vi "VIAn_CheckBrokenVIs.vi"(8 "error in (no error)":errorcluster, 11 "CommandLine":string[](array[string])) -> (0 "error out":errorcluster, 2 "test details":string, 3 "output to action":string)   [LabVIEW 2014]
uses:
  <userlib>/_OpenG.lib/string/string.llb/Trim Whitespace (String)__ogtk.vi
  <userlib>/_OpenG.lib/file/file.llb/File Exists - Scalar__ogtk.vi
  <userlib>/_OpenG.lib/array/array.llb/Filter 1D Array with Scalar (String)__ogtk.vi
  <userlib>/_OpenG.lib/array/array.llb/Empty 1D Array (String)__ogtk.vi
  <userlib>/_OpenG.lib/file/file.llb/Compare Two Paths - Scalar__ogtk.vi
  _lvcicd/_lvcicd_support_2014.lvlib
  <vilib>/addons/analyzer/NI_VIAnalyzerTKVIs.lvlib
panel:
  out "Analysis Progress":dbl(slide) scale=0.0..100.0
  out "VI in Analysis":string
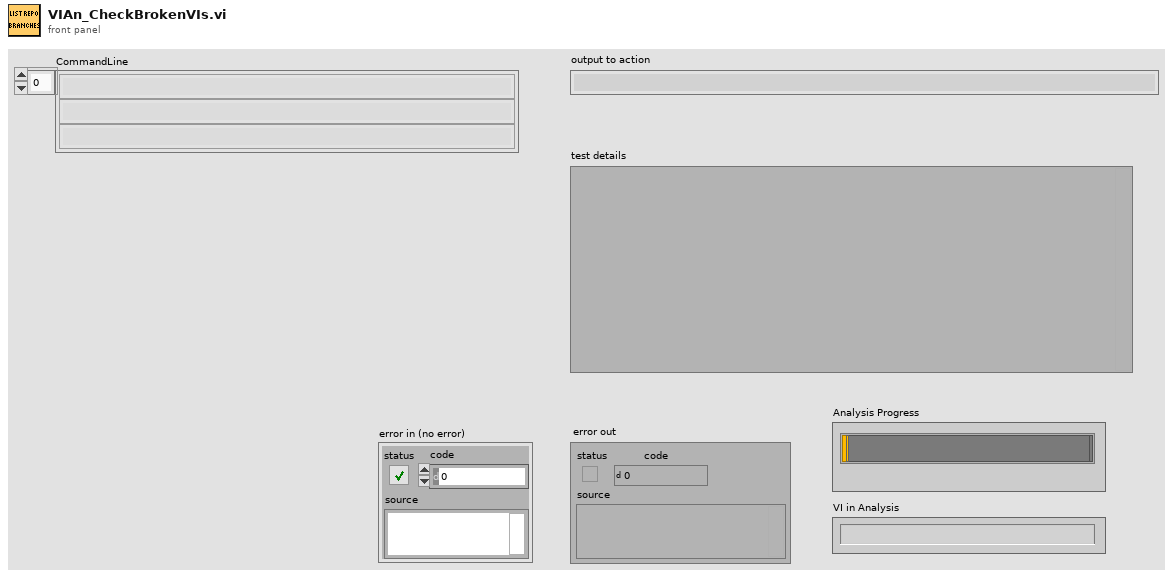
[diagram p1: front panel]
types:
  T1 = typedef "VIAnAPI Ref.ctl" = refnum<k1>
  T2 = typedef "VIAnCtl API Test Config Data.ctl" = cluster{"Test Ranking":T3, "Max Failures":u32, "Control Values":T4[], "Run Test?":bool}
  T3 = typedef "VIAnCtl TestRanking.ctl" = u16
  T4 = typedef "VIAnCtl Config Control Value.ctl" = cluster{"Control Name":string, "Control Value":variant}
  T5 = typedef "VIAnCtl Results.ctl" = cluster{"Test Name":string, "Results Data":T6[], "Status":T7, "Exceed Max Fails?":bool}
  T6 = typedef "VIAnCtl ResultsData (index).ctl" = cluster{"Result Message":string, "Ref Index":i32}
  T7 = typedef "VIAnCtl ResultStatus.ctl" = enum16{"Pass", "Fail", "Skipped", "VI not loadable", "Test not loadable", "Test not runnable", "Test error out"}
  T8 = typedef "VIAnRes Parsed Results Data (by VI).ctl" = cluster{"VI Path":path, "Pass":cluster{"row":i32, "column":i32}[], "Fail":cluster{"row":i32, "column":i32}[], "Skipped":cluster{"row":i32, "column":i32}[], "VI not loadable":cluster{"row":i32, "column":i32}[], "Test not loadable":cluster{"row":i32, "column":i32}[], "Test not runnable":cluster{"row":i32, "column":i32}[], "Test error out":cluster{"row":i32, "column":i32}[]}
  T9 = typedef "VIAnRes Parsed Results Data (by Test).ctl" = cluster{"Test Name":string, "Pass":cluster{"VI Path":path, "index":cluster{"row":i32, "column":i32}}[], "Fail":cluster{"VI Path":path, "index":cluster{"row":i32, "column":i32}}[], "Skipped":cluster{"VI Path":path, "index":cluster{"row":i32, "column":i32}}[]}
  T10 = typedef "VIAnCtl Test Config Data.ctl" = cluster{"Test Name":string, "Config Ref":refnum<vi>, "Ref Valid?":bool, "Test Ranking":T3, "Max Failures":u32, "Test Path":path, "Control Values":T4[], "Selected?":bool}
  T11 = cluster{"Raw Results":T5[][], "Parsed Results Data (by VI)":T8[], "Parsed Results Data (by Test)":T9[], "Summary Statistics":cluster{"Passed Tests":i32, "Failed Tests":i32, "Skipped Tests":i32, "VIs not loadable":i32, "Tests not loadable":i32, "Tests not runnable":i32, "Test error out":i32, "Start Time":u32, "Total Time (s)":dbl}, "Test Config Data":T10[]}
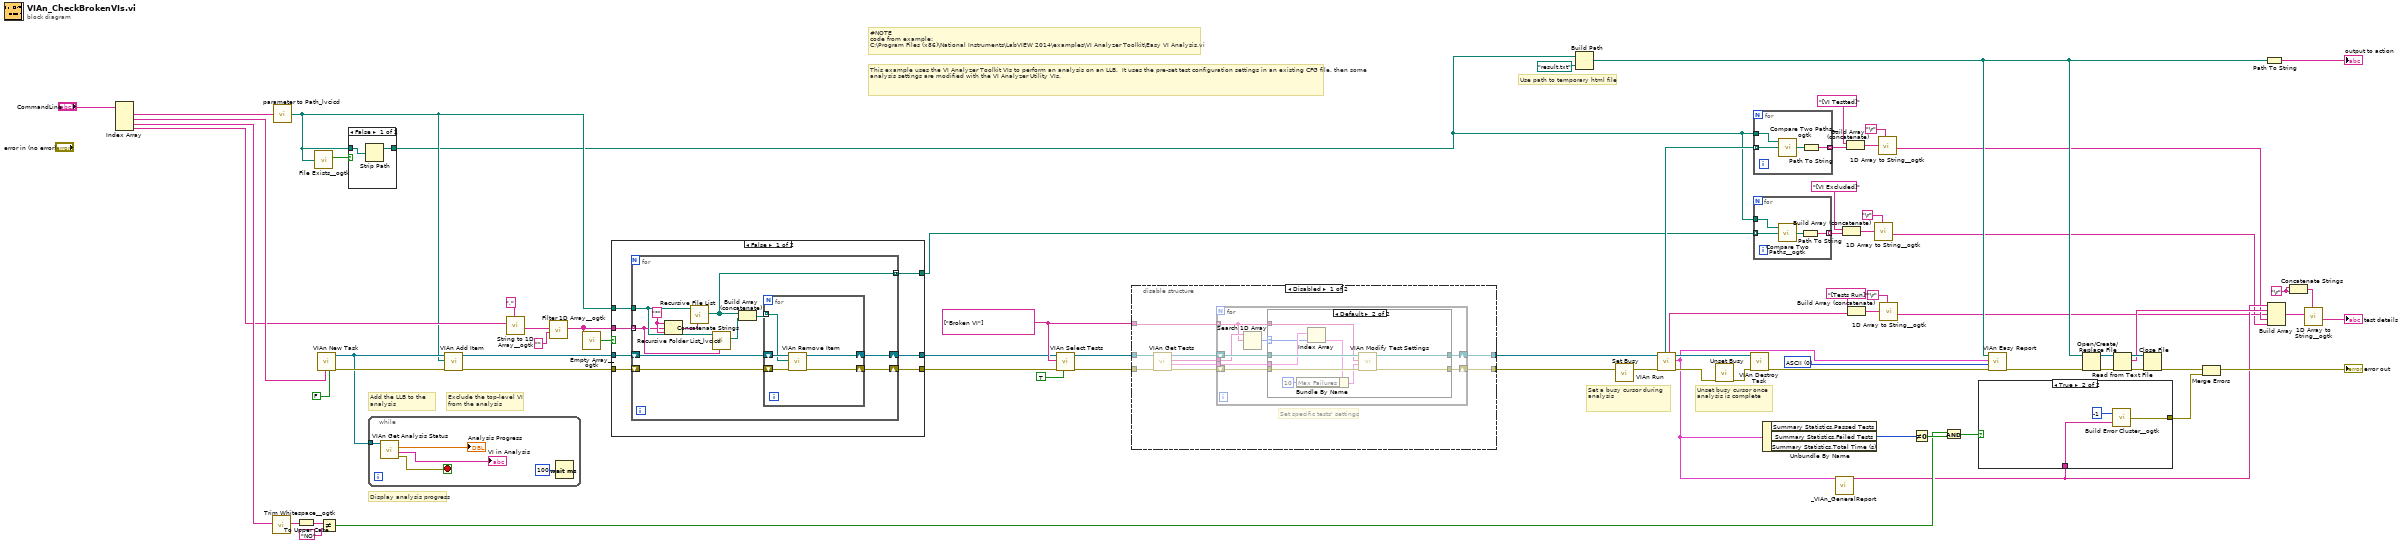
[diagram p0: block diagram]
diagram:
  w34 = "\r"
  w52 = string[] ["Broken VI"] ("Excluded Tests")
  w61 = u16 0 items=["ASCII", "HTML", "RSL File"] ("Report Save Type (ASCII)")
  # "Display analysis progress"
  # "Unset busy cursor once analysis is complete"
  # "Set a busy cursor during analysis"
  # "This example uses the VI Analyzer Toolkit VIs to perform an analysis on an LLB.  It uses the pre-set test configuration settings in an existing CFG file, then some analysis settings are modified with the VI Analyzer Utility VIs."
  # "Exclude the top-level VI from the analysis"
  # "Add the LLB to the analysis"
  # "#NOTE\ncode from example: \nC:\\Program Files (x86)\\National Instruments\\LabVIEW 2014\\examples\\VI Analyzer Toolkit\\Easy VI Analysis.vi"
  # "Use path to temporary html file"
  n1 = Index Array(array="CommandLine") -> (element #1=w73:string, element #2=w21:string, element #3=w22:string, element #4=w16:string)  [unwired: 4 in]
  n2 = call-poly <userlib>:"Trim Whitespace__ogtk.vi"("String in"=w22) -> ("String out"=w25:string)  [unwired: 6 in]
  n3 = call "parameter to Path_lvcicd.vi"("String"=w73) -> ("Path"=w14:path)
  n4 = To Upper Case(1:w25) -> (0:w26:string)
  n5 = call-poly <userlib>:"File Exists__ogtk.vi"("file path"=w14) -> ("is directory"=w51:bool)  [unwired: 6 in, 1 out]
  n6 = call <vilib>:"VIAn New Task.vi"("Select All Tests? (T)"=FALSE, "Configuration File Password"=w21) -> ("error out"=w64:errorcluster, "VI Analyzer Task out"=w56:T1)  [unwired: 2 in, 6 out]
  n7 = Not Equal?(x=w26, y="NO") -> (x != y?=w24:bool)
  n8 = case shown="False" w51 {
    tunnel: w14 -> [w75 w77]
    tunnel: [w76 w77] -> w2
    frame False {
      n9 = Strip Path(path=w75) -> (stripped path=w76:path)  [unwired: 1 out]
    }
    frame True {
    }
  }
  n10 = while {
    tunnel: w56 -> [w82]
    stop <- w78 stop-if-true
    n11 = call <vilib>:"VIAn Get Analysis Status.vi"("VI Analyzer Task in"=w82) -> ("error out"=w78:errorcluster, "VI in Analysis"=→"VI in Analysis":string, "Percent Complete"=→"Analysis Progress":dbl)  [unwired: 1 in, 7 out]
    n12 = Wait (ms)(milliseconds to wait=u32 100) -> ()  [unwired: 1 out]
  }
  n13 = call <vilib>:"VIAn Add Item.vi"("error in (no error)"=w64, "Item to Add"=w14, "VI Analyzer Task in"=w56) -> ("error out"=w19:errorcluster, "VI Analyzer Task out"=w20:T1)  [unwired: 7 out]
  n14 = call <userlib>:"String to 1D Array__ogtk.vi"("delimiter (Tab)"=",", "string"=w16) -> ("Array of Strings"=w12:string[])  [unwired: 9 in]
  n15 = call-poly <userlib>:"Filter 1D Array__ogtk.vi"("items to filter"="" ("delimiter (Tab)"), "array"=w12) -> ("filtered array"=w11:string[])  [unwired: 4 in, 1 out]
  n16 = call-poly <userlib>:"Empty Array__ogtk.vi"("Array"=w11) -> ("Empty Array?"=w13:bool)  [unwired: 8 in]
  n17 = case shown="False" w13 {
    tunnel: w20 -> [w89 w107]
    tunnel: w19 -> [w88 w106]
    tunnel: [w87 w107] -> w18
    tunnel: [w86 w106] -> w17
    tunnel: w11 -> [w85 _]
    tunnel: w14 -> [w84 _]
    tunnel: [w83 _] -> w3
    frame False {
      n18 = for {
        tunnel: w84 -> [w93]
        shift-right: [w98] -> w87
        shift-left: w89 -> [w100]
        shift-right: [w97] -> w86
        shift-left: w88 -> [w99]
        tunnel: w85 -> [w92] mode=indexing
        tunnel: [w94] -> w83 mode=concatenating
        w95 = "*" ("string")
        n19 = Concatenate Strings(w95, w92, w95) -> (w96:string)
        n20 = call <vilib>:"Recursive File List.vi"("pattern"=w96, "Folder Path"=w93) -> ("All Files in Dir"=w94:path[])  [unwired: 5 in, 4 out]
        n21 = call "Recursive Folder List_lvcicd.vi"("pattern"=w92, "Folder Path"=w93) -> ("All Folders"=w90:path[])  [unwired: 6 in, 3 out]
        n22 = Build Array (concatenate)(w94, w90) -> (w91:path[])
        n23 = for {
          tunnel: w91 -> [w101] mode=indexing
          shift-right: [w103] -> w98
          shift-left: w100 -> [w105]
          shift-right: [w102] -> w97
          shift-left: w99 -> [w104]
          n24 = call <vilib>:"VIAn Remove Item.vi"("error in (no error)"=w104, "Item to Remove"=w101, "VI Analyzer Task in"=w105) -> ("error out"=w102:errorcluster, "VI Analyzer Task out"=w103:T1)  [unwired: 7 out]
        }
      }
    }
    frame True {
    }
  }
  n25 = call <vilib>:"VIAn Select Tests.vi"("Select Test? (T)"=TRUE, "error in (no error)"=w17, "Test Names"=w52, "VI Analyzer Task in"=w18) -> ("error out"=w53:errorcluster, "VI Analyzer Task out"=w54:T1)  [unwired: 6 out]
  n26 = disable-structure shown="Disabled" {
    disable-tunnel: [w116 w138] -> w60
    disable-tunnel: [w115 w137] -> w59
    disable-tunnel: w54 -> [w114 w138]
    disable-tunnel: w53 -> [w113 w137]
    disable-tunnel: w52 -> [w108 _]
    frame Disabled {
      # "Set specific tests' settings"
      n27 = call <vilib>:"VIAn Get Tests.vi"("error in (no error)"=w113, "VI Analyzer Task in"=w114) -> ("error out"=w112:errorcluster, "Test Configurations"=w110:T2[], "Test Names"=w109:string[], "VI Analyzer Task out"=w111:T1)  [unwired: 6 out]
      n28 = for {
        shift-right: [w121] -> w115
        shift-left: w112 -> [w123]
        shift-right: [w122] -> w116
        shift-left: w111 -> [w124]
        tunnel: w108 -> [w119] mode=indexing
        tunnel: w110 -> [w117]
        tunnel: w109 -> [w120]
        n29 = Search 1D Array(1D array=w120, element=w119) -> (index of element=w118:i32)  [unwired: 1 out]
        n30 = case shown="Default" w118 {
          selector: w118 -> [_ w129]
          tunnel: w124 -> [w126 w136]
          tunnel: w123 -> [w125 w135]
          tunnel: [w126 w134] -> w122
          tunnel: [w125 w133] -> w121
          tunnel: w119 -> [_ w131]
          tunnel: w117 -> [_ w130]
          frame -1 {
          }
          frame Default {
            n31 = Index Array(array=w130, index=w129) -> (element=w128:T2)
            n32 = Bundle By Name(cluster=w128, "Max Failures"=u32 10) -> (w132:T2)
            n33 = call <vilib>:"VIAn Modify Test Settings.vi"("error in (no error)"=w135, "New Test Info"=w132, "Test Name"=w131, "VI Analyzer Task in"=w136) -> ("error out"=w133:errorcluster, "VI Analyzer Task out"=w134:T1)  [unwired: 6 out]
          }
        }
      }
    }
    frame Enabled {
    }
  }
  n34 = Build Path(base path=w2, name or relative path=path "result.txt" ("path")) -> (appended path=w49:path)
  n35 = call <vilib>:"Set Busy.vi"("error in (no error)"=w59) -> ("error out"=w58:errorcluster)  [unwired: 3 in, 7 out]
  n36 = call <vilib>:"VIAn Run.vi"("error in (no error)"=w58, "VI Analyzer Task in"=w60) -> ("error out"=w50:errorcluster, "Analysis Results"=w28:T11, "VI Analyzer Task out"=w63:T1, "Tests Run"=w39:string[], "VIs Tested"=w47:path[])  [unwired: 5 out]
  n37 = call <vilib>:"Unset Busy.vi"("error in (no error)"=w50) -> ("error out"=w57:errorcluster)  [unwired: 1 in, 9 out]
  n38 = call <vilib>:"VIAn Destroy Task.vi"("error in (no error)"=w57, "VI Analyzer Task in"=w63) -> ("error out"=w62:errorcluster)  [unwired: 9 out]
  n39 = for {
    tunnel: w3 -> [w139] mode=indexing
    tunnel: w2 -> [w140]
    tunnel: [w141] -> w6 mode=indexing
    n40 = call-poly <userlib>:"Compare Two Paths__ogtk.vi"("path2"=w139, "path1"=w140) -> ("relative path from 1 to 2"=w142:path)  [unwired: 1 in, 2 out]
    n41 = Path To String(path=w142) -> (string=w141:string)
  }
  n42 = for {
    tunnel: w47 -> [w143] mode=indexing
    tunnel: w2 -> [w144]
    tunnel: [w145] -> w46 mode=indexing
    n43 = call-poly <userlib>:"Compare Two Paths__ogtk.vi"("path2"=w143, "path1"=w144) -> ("relative path from 1 to 2"=w146:path)  [unwired: 1 in, 2 out]
    n44 = Path To String(path=w146) -> (string=w145:string)
  }
  n45 = Unbundle By Name(w28) -> ("Summary Statistics.Failed Tests"=w29:i32)  [unwired: 2 out]
  n46 = call "_VIAn_GeneralReport.vi"("Analysis Results"=w28) -> ("String"=w23:string)  [unwired: 7 in, 3 out]
  n47 = Build Array (concatenate)("[VI Excluded]" ("string"), w6) -> (w8:string[])
  n48 = Build Array (concatenate)("[VI Testted]" ("string"), w46) -> (w44:string[])
  n49 = Build Array (concatenate)("[Tests Run]" ("string"), w39) -> (w41:string[])
  n50 = call <userlib>:"1D Array to String__ogtk.vi"("delimiter (Tab)"="\r", "Array of Strings"=w8) -> ("delimited string"=w1:string)  [unwired: 9 in]
  n51 = call <userlib>:"1D Array to String__ogtk.vi"("delimiter (Tab)"="\r", "Array of Strings"=w44) -> ("delimited string"=w5:string)  [unwired: 9 in]
  n52 = call <userlib>:"1D Array to String__ogtk.vi"("delimiter (Tab)"="\r", "Array of Strings"=w41) -> ("delimited string"=w4:string)  [unwired: 9 in]
  n53 = Not Equal To 0?(x=w29) -> (x != 0?=w31:bool)
  n54 = And(x=w24, y=w31) -> (x .and. y?=w30:bool)
  n55 = case shown="True" w30 {
    tunnel: [_ w148] -> w32
    tunnel: w23 -> [_ w147]
    frame False {
    }
    frame True {
      n56 = call <userlib>:"Build Error Cluster__ogtk.vi"("String to Prepend to source (\"\")"=w147, "code"=-1) -> ("error out"=w148:errorcluster)
    }
  }
  n57 = call <vilib>:"VIAn Easy Report.vi"("error in (no error)"=w62, "Report Save Type (ASCII)"=w61, "Analysis Results"=w28, "Report Save Path"=w49) -> ("error out"=w48:errorcluster)  [unwired: 3 in, 4 out]
  n58 = Open/Create/Replace File(file path (use dialog)=w49, error in=w48) -> (refnum out=w67:refnum<file>, error out=w69:errorcluster)  [unwired: 4 in, 1 out]
  n59 = Read from Text File(file (use dialog)=w67, error in=w69) -> (refnum out=w66:refnum<file>, text=w33:string, error out=w68:errorcluster)  [unwired: 2 in, 1 out]
  n60 = Close File(refnum=w66, error in=w68) -> (error out=w70:errorcluster)  [unwired: 1 out]
  n61 = Merge Errors(w70, w32) -> (→"error out":errorcluster)
  n62 = Path To String(path=w49) -> (string=→"output to action":string)
  n63 = Build Array(w23, w33, w4, w5, w1) -> (w37:string[])
  n64 = Concatenate Strings(w34, w34) -> (w35:string)
  n65 = call <userlib>:"1D Array to String__ogtk.vi"("delimiter (Tab)"=w35, "Array of Strings"=w37) -> ("delimited string"=→"test details":string)  [unwired: 9 in]
